vi "2 Area of Triangle.vi"(9 "pt C":T1 {"North" format="%#_10f"; "East" format="%#_8f"}, 10 "pt B":T1 {"North" format="%#_10f"; "East" format="%#_8f"}, 11 "pt A":T1 {"North" format="%#_10f"; "East" format="%#_8f"}) -> (2 "Area":dbl)   [LabVIEW 2011]
doc: "Uses math found here: http://people.richland.edu/james/lecture/m116/matrices/area.html to determine the area of a triangle"
uses:
  2 Typedefs/UTM Location.ctl
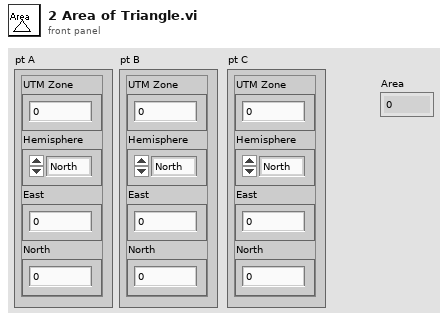
[diagram p1: front panel]
types:
  T1 = typedef "UTM Location.ctl" = cluster{"UTM Zone":dbl, "Hemisphere":enum16{"North", "South"}, "East":dbl, "North":dbl}
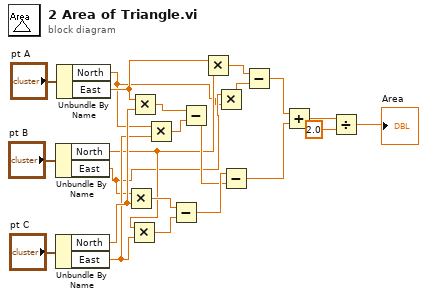
[diagram p0: block diagram]
diagram:
  n1 = Unbundle By Name("pt B") -> ("North"=w10:dbl, "East"=w7:dbl)
  n2 = Unbundle By Name("pt C") -> ("North"=w17:dbl, "East"=w16:dbl)
  n3 = Unbundle By Name("pt A") -> ("North"=w6:dbl, "East"=w11:dbl)
  n4 = Multiply(x=w7, y=w17) -> (x*y=w19:dbl)
  n5 = Multiply(x=w10, y=w16) -> (x*y=w18:dbl)
  n6 = Multiply(x=w11, y=w17) -> (x*y=w15:dbl)
  n7 = Multiply(x=w6, y=w16) -> (x*y=w14:dbl)
  n8 = Subtract(x=w19, y=w18) -> (x-y=w13:dbl)
  n9 = Subtract(x=w15, y=w14) -> (x-y=w12:dbl)
  n10 = Multiply(x=w11, y=w10) -> (x*y=w9:dbl)
  n11 = Multiply(x=w7, y=w6) -> (x*y=w8:dbl)
  n12 = Subtract(x=w13, y=w12) -> (x-y=w4:dbl)
  n13 = Subtract(x=w9, y=w8) -> (x-y=w5:dbl)
  n14 = Add(x=w5, y=w4) -> (x+y=w3:dbl)
  n15 = Divide(x=w3, y=2.0) -> (x/y=→"Area":dbl)
